vi "Read retries.vi"(8 "error in (no error)":errorcluster, 11 "MB_Master_Serial in":refnum<class "MB_Master_Serial.lvclass">) -> (0 "error out":errorcluster, 2 "retries":i32=1, 3 "MB_Master_Serial out":refnum<class "MB_Master_Serial.lvclass">)   [LabVIEW 2016, in "MB Master.lvlib" / "MB_Master_Serial.lvclass"]
uses:
  MB_Master_Serial.lvclass
  MB_Master_Serial.lvclass/MB_Master_Serial.ctl
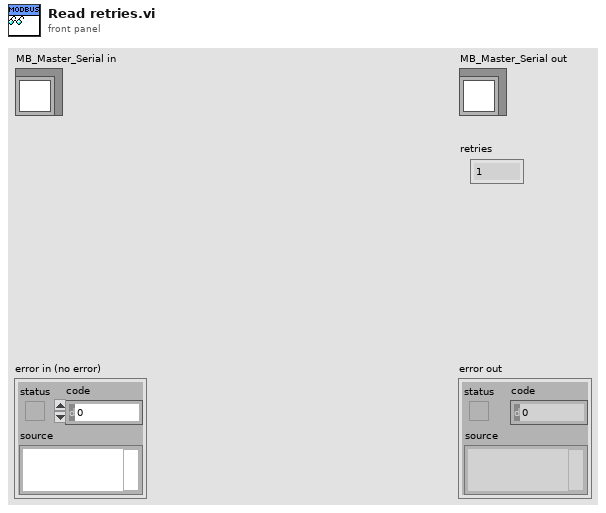
[diagram p1: front panel]
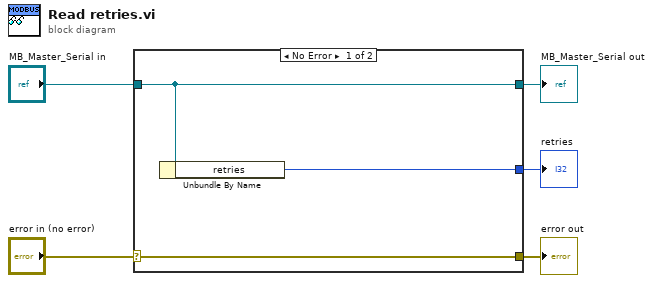
[diagram p0: block diagram]
diagram:
  n1 = case shown="No Error" "error in (no error)" {
    selector: "error in (no error)" -> [w8 w9]
    tunnel: [w8 w9] -> w4
    tunnel: [w7 w10] -> w2
    tunnel: "MB_Master_Serial in" -> [w7 w10]
    tunnel: [w6 _] -> w1
    frame No Error {
      n2 = Unbundle By Name(w7) -> ("retries"=w6:i32)
    }
    frame Error {
    }
  }
  "error out" <- w4
  "MB_Master_Serial out" <- w2
  "retries" <- w1
